vi "DatabaseLab.vi"() -> ()   [LabVIEW 2021]
uses:
  <vilib>/numeric/Random Number (Range) U64.vi
  <vilib>/numeric/sub_Random U32.vi
panel:
  out "Current Average in Living Room":string[][](array[string])
  out "Storage Procedure being sent to SQL":string
  out "Sensor being Sampled":dbl
  in  "stop":bool
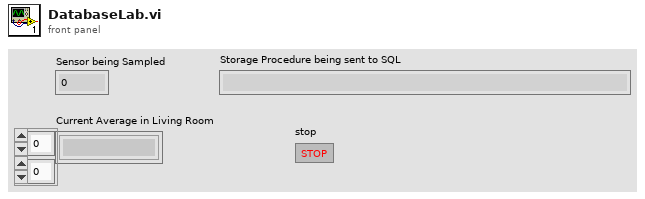
[diagram p1: front panel]
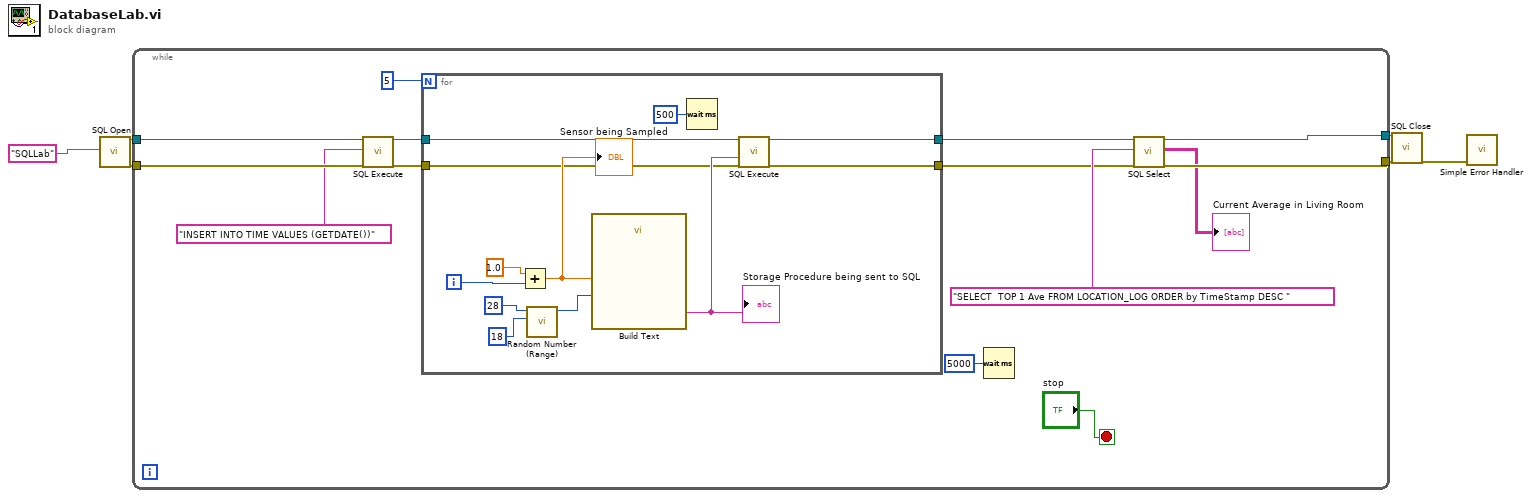
[diagram p0: block diagram]
diagram:
  n1 = call "SQL Open.vi"("ConnectionString In"="SQLLab") -> ("Connection Out"=w4:refnum<k7>, "Error out"=w5:errorcluster)  [unwired: 17 in]
  n2 = while {
    tunnel: w5 -> [w16]
    tunnel: w4 -> [w17]
    tunnel: [w9] -> w3
    tunnel: [w8] -> w2
    stop <- "stop" stop-if-true
    n3 = call "SQL Execute.vi"("Connection In"=w17, "SQL Query"="INSERT INTO TIME VALUES (GETDATE())", "Error in (no error)"=w16) -> ("Connection Out"=w15:refnum<k7>, "Error out"=w14:errorcluster)  [unwired: 15 in]
    n4 = for {
      N: 5 -> [_]
      tunnel: w14 -> [w23]
      tunnel: w15 -> [w24]
      tunnel: [w22] -> w10
      tunnel: [w21] -> w11
      i -> [w27]
      n5 = Add(x=1.0, y=w27) -> (x+y=w26:dbl)
      "Sensor being Sampled" <- w26
      n6 = call-poly <vilib>:"Random Number (Range).vi"("lower bound (0)"=u64 18, "upper bound (100)"=u64 28) -> ("number"=w29:u64)  [unwired: 9 in]
      n7 = call "Build Text"("Sensor"=w26, "Value"=w29) -> ("Result"=w25:string)  [unwired: 12 in, 1 out]
      "Storage Procedure being sent to SQL" <- w25
      n8 = Wait (ms)(milliseconds to wait=u32 500) -> ()  [unwired: 1 out]
      n9 = call "SQL Execute.vi"("Connection In"=w24, "SQL Query"=w25, "Error in (no error)"=w23) -> ("Connection Out"=w22:refnum<k7>, "Error out"=w21:errorcluster)  [unwired: 15 in]
    }
    n10 = Wait (ms)(milliseconds to wait=u32 5000) -> ()  [unwired: 1 out]
    n11 = call "SQL Select.vi"("Connection In"=w10, "SQL Query"="SELECT  TOP 1 Ave FROM LOCATION_LOG ORDER by TimeStamp DESC ", "Error in (no error)"=w11) -> ("Connection Out"=w9:refnum<k7>, "Data"=→"Current Average in Living Room":string[][], "Error out"=w8:errorcluster)  [unwired: 14 in]
  }
  n12 = call "SQL Close.vi"("Connection In"=w3, "Error in (no error)"=w2) -> ("Error out"=w1:errorcluster)  [unwired: 17 in]
  n13 = call <vilib>:"Simple Error Handler.vi"("error in (no error)"=w1) -> ()  [unwired: 4 in, 5 out]
